vi "add percentage(SubVI).vi"(4 "y%":dbl, 5 "x":dbl) -> (1 "x(1+0.01y)":dbl)   [LabVIEW 2024]
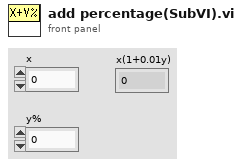
[diagram p1: front panel]
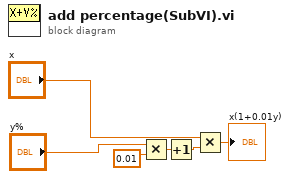
[diagram p0: block diagram]
diagram:
  n1 = Multiply(x="y%", y=0.01) -> (x*y=w5:dbl)
  n2 = Increment(x=w5) -> (x+1=w4:dbl)
  n3 = Multiply(x="x", y=w4) -> (x*y=→"x(1+0.01y)":dbl)
